vi "Path_Creator.vi"(0 "Raw_File_Path_In":path, 1 "VDDA":dbl, 2 "VDD":dbl, 3 "IMULT":dbl, 5 "SNR_Plot_Path":path, 7 "Temp":dbl, 9 "ADC_Controls":T2={"ACQPS"=12, "Break_PT"=0, "Ref_Mod_Sel"=enum."Int_Ref_2P5", "Ref_Sel(Int/Ext)"=enum."Ext", "ADC"=enum."A", "Channel"=0, "LV_samples"=8192, "AGPIO_SEL"=0.0, "LV_perscale"=2}, 11 "Repeat":dbl) -> (4 "Raw_File_Path_Out":path, 6 "SNR_File_Path_out":path)   [LabVIEW 2019]
uses:
  Ctrls/ADC_CTRL.ctl
panel:
  out "resulting string":string
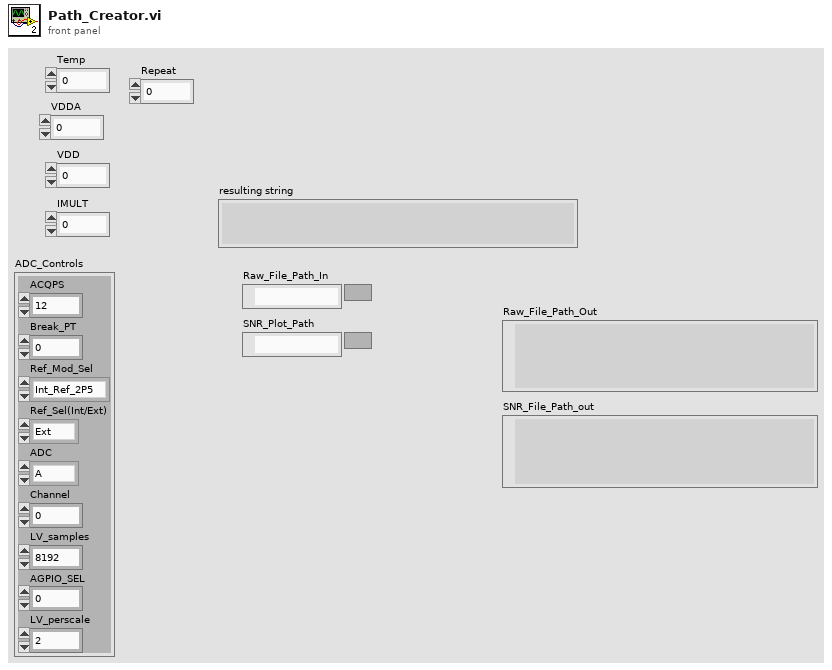
[diagram p1: front panel]
types:
  T1 = typedef "ADC_CTRL.ctl" = enum16{"A", "B", "C"}
  T2 = cluster{"ACQPS":u16, "Break_PT":u16, "Ref_Mod_Sel":enum16{"Int_Ref_1P65", "Int_Ref_2P5"}, "Ref_Sel(Int/Ext)":enum16{"Int", "Ext"}, "ADC":T1, "Channel":u16, "LV_samples":u16, "AGPIO_SEL":dbl, "LV_perscale":u16}
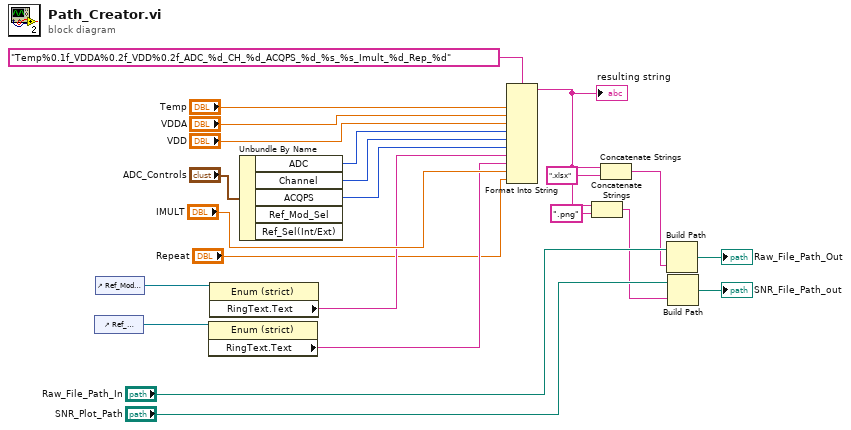
[diagram p0: block diagram]
diagram:
  n1 = control-ref of="Ref_Sel(Int/Ext)"() -> (w12:refnum<vi>)
  n2 = control-ref of="Ref_Mod_Sel"() -> (w14:refnum<vi>)
  n3 = property class="Enum (strict)"(reference=w12) -> ("RingText.Text"=w11:string)  [unwired: 1 in, 2 out]
  n4 = property class="Enum (strict)"(reference=w14) -> ("RingText.Text"=w13:string)  [unwired: 1 in, 2 out]
  n5 = Unbundle By Name("ADC_Controls") -> ("ADC"=w18:T1, "Channel"=w17:u16, "ACQPS"=w16:u16)  [unwired: 2 out]
  n6 = Format Into String(format string="Temp%0.1f_VDDA%0.2f_VDD%0.2f_ADC_%d_CH_%d_ACQPS_%d_%s_%s_Imult_%d_Rep_%d", "Temp", "VDDA", "VDD", w18, w17, w16, w13, w11, "IMULT", "Repeat") -> (resulting string=w8:string)  [unwired: 2 in, 1 out]
  "resulting string" <- w8
  n7 = Concatenate Strings(w8, ".png" ("string")) -> (w5:string)
  n8 = Concatenate Strings(w8, ".xlsx" ("string")) -> (w6:string)
  n9 = Build Path(base path="Raw_File_Path_In", name or relative path=w6) -> (appended path=→"Raw_File_Path_Out":path)
  n10 = Build Path(base path="SNR_Plot_Path", name or relative path=w5) -> (appended path=→"SNR_File_Path_out":path)
